vi "TagDB-Read As Variant.vi"(8 "error in (no error)":errorcluster, 10 "name":string, 11 "TagContainer":T1) -> (0 "error out":errorcluster, 1 "found":bool, 2 "Value":variant, 3 "TagContainer(dup)":T1, 4 "Time Stamp":timestamp, 5 "Raw name":string)   [LabVIEW 2017, in "TagDB(DEV).lvlib"]
uses:
  TagDB(DEV).lvlib
  Typedef/TagContainer.ctl
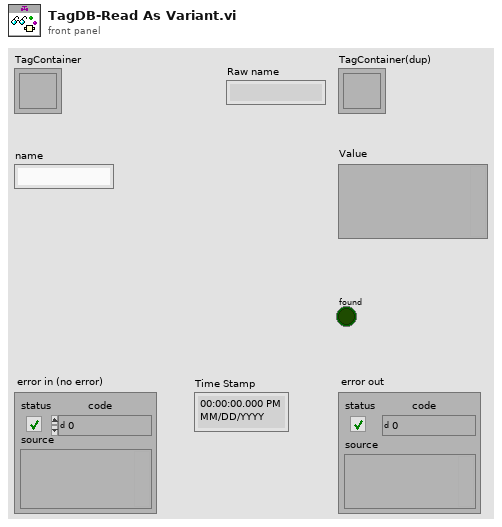
[diagram p1: front panel]
types:
  T1 = typedef "TagDB(DEV).lvlib/TagContainer.ctl" = refnum<k1>
  T2 = typedef "TagContainer(DEV).lvlib/tagcontainer-data.ctl" = cluster{"tag-map":variant, "timestamp-map":variant, "namecacher-map":variant, "DataTypeCacher-map":variant, "Tag Adding Lock?":bool, "Global Change Timestamp":timestamp, "Item Change Timestamp":timestamp, "name":string}
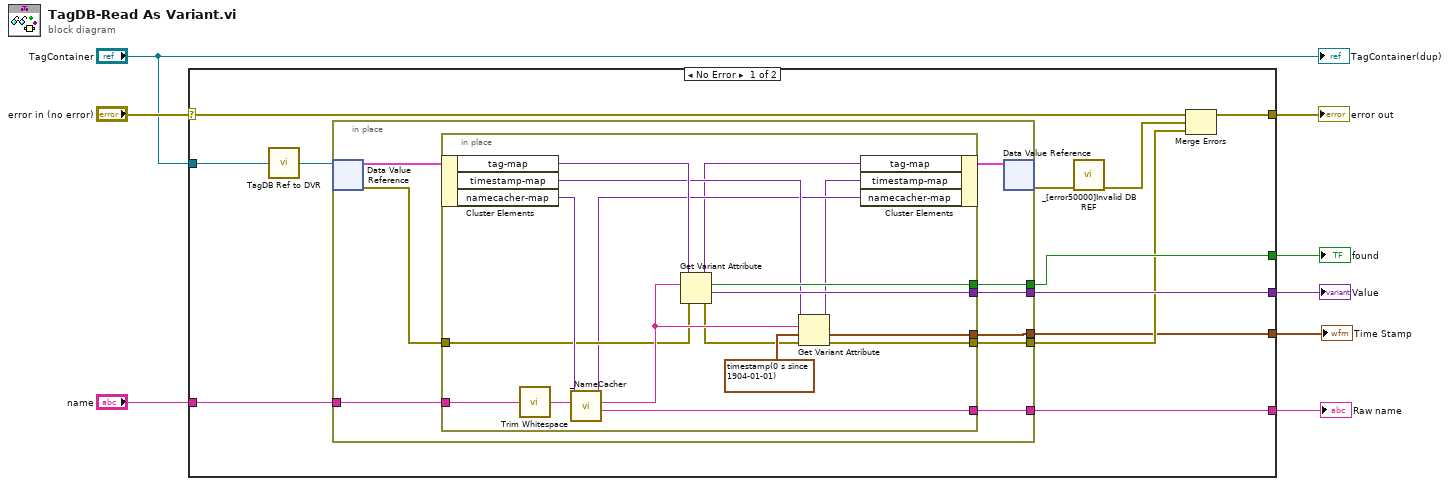
[diagram p0: block diagram]
diagram:
  n1 = case shown="No Error" "error in (no error)" {
    selector: "error in (no error)" -> [w19 w47]
    tunnel: [w20 w47] -> w7
    tunnel: "TagContainer" -> [w18 _]
    tunnel: [w17 _] -> w6
    tunnel: [w16 _] -> w5
    tunnel: [w13 _] -> w3
    tunnel: "name" -> [w12 _]
    tunnel: [w11 _] -> w1
    frame No Error {
      n2 = call "TagDB Ref to DVR.vi"("TagDB"=w18) -> ("DVR"=w15:refnum<data-value>)  [unwired: 4 in]
      n3 = in-place "In Place Element Structure" {
        in-place-border: [w29] -> w17
        in-place-border: [w28] -> w16
        in-place-border: [w27] -> w14
        in-place-border: [w26] -> w13
        in-place-border: w12 -> [w25]
        in-place-border: [w24] -> w11
        n4 = in-place-dvr #1(w15) -> (w23:T2, w21:errorcluster)
        n5 = in-place {
          in-place-border: [w46] -> w29
          in-place-border: [w45] -> w28
          in-place-border: [w43] -> w27
          in-place-border: [w42] -> w26
          in-place-border: w25 -> [w40]
          in-place-border: [w39] -> w24
          in-place-border: w21 -> [w34]
          n6 = in-place-cluster #2(w23) -> ("tag-map"=w37:variant, "timestamp-map"=w36:variant, "namecacher-map"=w35:variant)
          n7 = call <vilib>:"Trim Whitespace.vi"("string"=w40) -> ("trimmed string"=w41:string)  [unwired: 1 in]
          n8 = call "_NameCacher.vi"("key"=w41, "cacher"=w35) -> ("Raw name"=w39:string, "Key in lower case"=w38:string, "cacher out"=w33:variant)  [unwired: 7 in]
          n9 = Get Variant Attribute(Variant=w37, name=w38, error in=w34) -> (duplicate Variant=w31:variant, found=w45:bool, value=w46:variant, error out=w32:errorcluster)  [unwired: 1 in]
          n10 = Get Variant Attribute(Variant=w36, name=w38, default value (empty Variant)=timestamp(0 s since 1904-01-01) ("Time Stamp"), error in=w32) -> (duplicate Variant=w30:variant, value=w42:timestamp, error out=w43:errorcluster)  [unwired: 1 out]
          n11 = in-place-cluster #2("tag-map"=w31, "timestamp-map"=w30, "namecacher-map"=w33) -> (w22:T2)
        }
        n12 = in-place-dvr #1(w22) -> (w10:errorcluster)  [unwired: 1 out]
      }
      n13 = call "_[error50000]Invalid DB REF.vi"("error in (no error)"=w10) -> ("error out"=w9:errorcluster)  [unwired: 10 in]
      n14 = Merge Errors(w19, w9, w14) -> (w20:errorcluster)
    }
    frame Error {
    }
  }
  "error out" <- w7
  "Value" <- w6
  "found" <- w5
  "Time Stamp" <- w3
  "Raw name" <- w1
  "TagContainer(dup)" <- "TagContainer"
